vi "Measurement Logic.vi"() -> ()   [LabVIEW 2021, in "DAQmx Continuous Voltage Input.lvlib"]
uses:
  DAQmx Continuous Voltage Input.lvlib
  Measurement Configuration.ctl
  Measurement Results.ctl
  <vilib>/MeasurementLink/MeasurementLink Measurement Server/Measure Call Context/Measure Call Context.lvclass
  <vilib>/Utility/error.llb/DialogType.ctl
  Typedef/Analog Start.ctl
  Typedef/Analog Pause.ctl
  Typedef/Waveform.ctl
  <vilib>/DAQmx/read.llb/DAQmx Read (Analog 1D Wfm NChan NSamp).vi
  <vilib>/DAQmx/create/channels.llb/DAQmx Create Channel (AI-Voltage-Basic).vi
  <vilib>/DAQmx/configure/timing.llb/DAQmx Timing (Sample Clock).vi
  <vilib>/DAQmx/configure/task.llb/DAQmx Configure Logging (TDMS).vi
  <vilib>/DAQmx/configure/trigger.llb/DAQmx Start Trigger (Digital Edge).vi
  <vilib>/DAQmx/configure/trigger.llb/DAQmx Start Trigger (Time).vi
  <vilib>/DAQmx/configure/trigger.llb/DAQmx Start Trigger (Analog Edge).vi
  <vilib>/DAQmx/miscellaneous.llb/DAQmx Fill In Error Info.vi
  <resource>/objmgr/daqmx.rc
panel:
  out "measure call context out":refnum<class "Measure Call Context.lvclass">
  in  "measure call context in":refnum<class "Measure Call Context.lvclass">
  out "measurement results":T1
  in  "measurement configuration":T2={"Max Voltage"=5.0, "Min Voltage"=-5.0, "Terminal Configuration"=-1, "Sample Rate"=1000.0, "Number of Samples"=100, "Logging Mode"=10231, "TDMS File Path"="", "Trigger Tab Enum"=enum."No Trigger", "Analog Start str"="", "Digital Start Source str"="", "Digital Pause Source str"="", "Digital Start Trigger Edge"=10280, "Digital Pause Trigger Pause When"=10192, "Physical Channel str"="Dev1/ai0", "Sample Clock Source str"="OnboardClock", "Select Time Manually"=FALSE, "When str"="", "Analog Pause str"=""} {"Digital Pause Trigger Pause When" items=["High"=10192, "Low"=10214]; "Digital Start Trigger Edge" items=["Rising"=10280, "Falling"=10171]; "Logging Mode" items=["Off"=10231, "Log and Read"=15842]; "Terminal Configuration" items=["default"=-1, "RSE"=10083, "NRSE"=10078, "Differential"=10106, "Pseudodifferential"=12529]}
  # "Source: LabVIEW - examples\\DAQmx\\Analog Input\\Voltage - Continuous Input.vi"
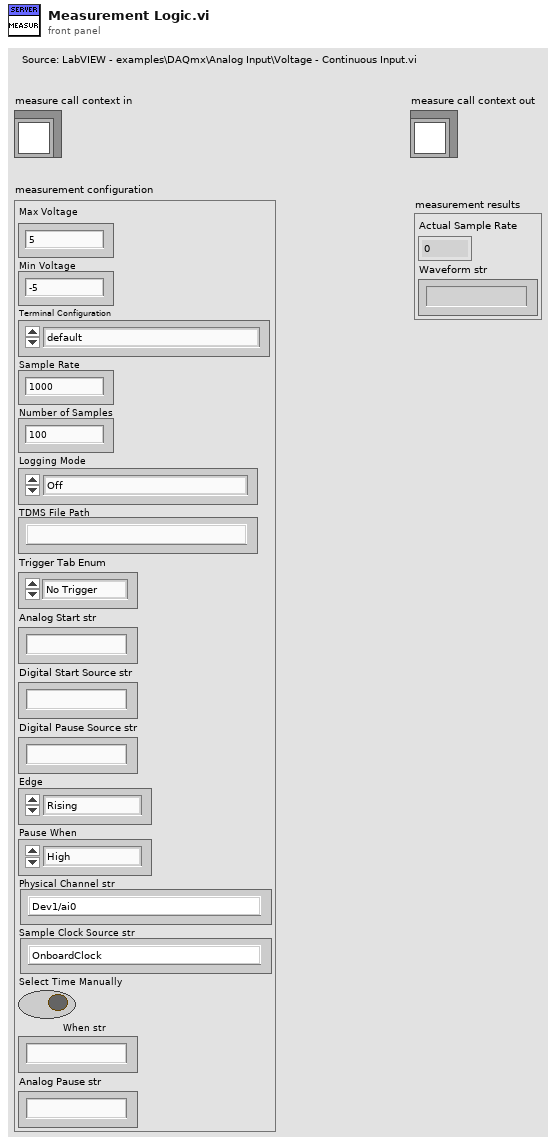
[diagram p1: front panel]
types:
  T1 = typedef "DAQmx Continuous Voltage Input.lvlib/Measurement Results.ctl" = cluster{"Actual Sample Rate":dbl, "Waveform str":string}
  T2 = typedef "DAQmx Continuous Voltage Input.lvlib/Measurement Configuration.ctl" = cluster{"Max Voltage":dbl, "Min Voltage":dbl, "Terminal Configuration":i32, "Sample Rate":dbl, "Number of Samples":i32, "Logging Mode":i32, "TDMS File Path":string, "Trigger Tab Enum":enum32{"No Trigger", "Digital Start", "Digital Pause", "Digital Reference", "Analog Start", "Analog Pause", "Analog Reference", "Time Start"}, "Analog Start str":string, "Digital Start Source str":string, "Digital Pause Source str":string, "Digital Start Trigger Edge":i32, "Digital Pause Trigger Pause When":i32, "Physical Channel str":string, "Sample Clock Source str":string, "Select Time Manually":bool, "When str":string, "Analog Pause str":string}
  T3 = typedef "DialogType.ctl" = u16
  T4 = enum32{"No Trigger", "Digital Start", "Digital Pause", "Digital Reference", "Analog Start", "Analog Pause", "Analog Reference", "Time Start"}
  T5 = typedef "DAQmx Continuous Voltage Input.lvlib/Analog Start.ctl" = cluster{"Analog Start Trigger Source":string, "Analog Start Trigger Slope":i32, "Analog Start Trigger Hysteresis":dbl, "Analog Start Trigger Level":dbl}
  T6 = typedef "DAQmx Continuous Voltage Input.lvlib/Analog Pause.ctl" = cluster{"Analog Pause Trigger Source":string, "Analog Pause Trigger Pause When":i32, "Analog Pause Trigger Level":dbl}
  T7 = typedef "DAQmx Continuous Voltage Input.lvlib/Waveform.ctl" = cluster{"Y":dbl[], "dt":dbl}
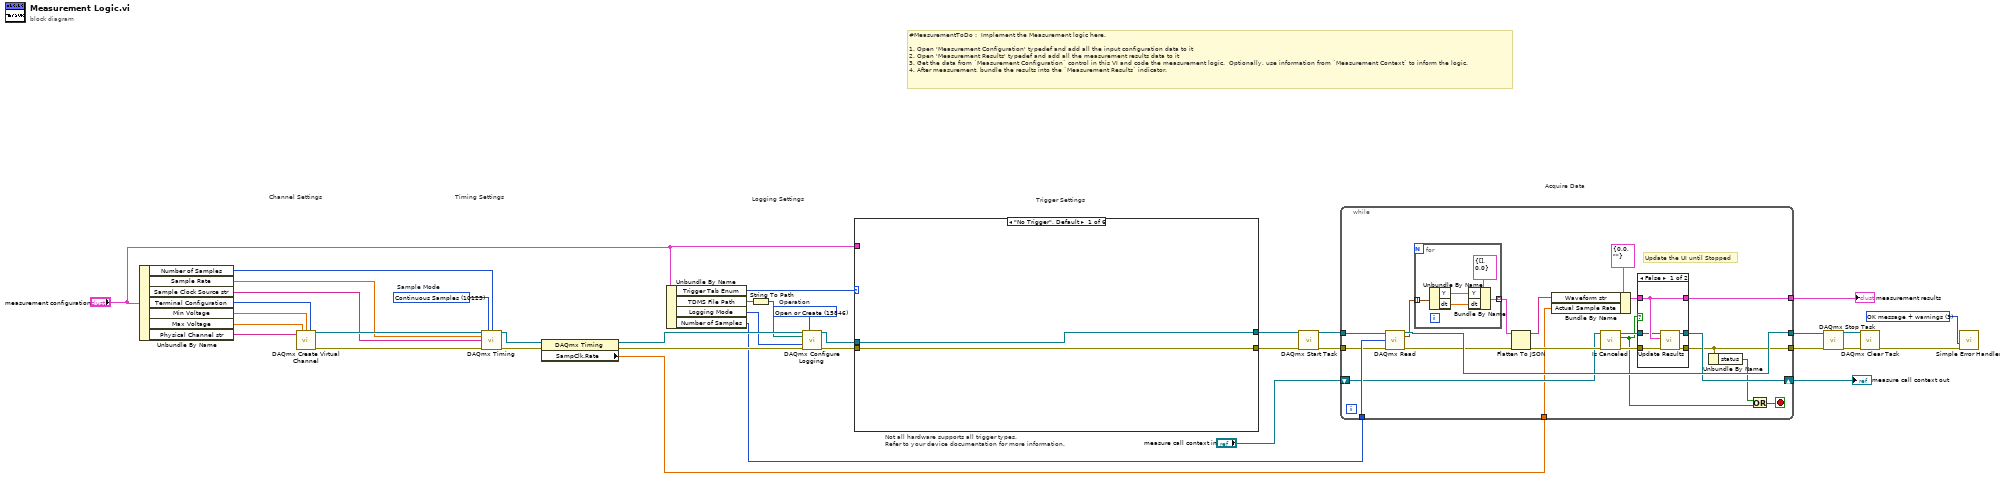
[diagram p0: block diagram]
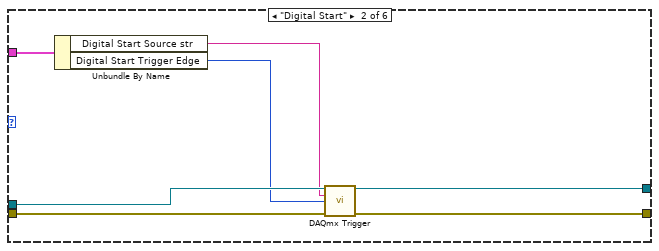
[diagram p2: hidden frame]
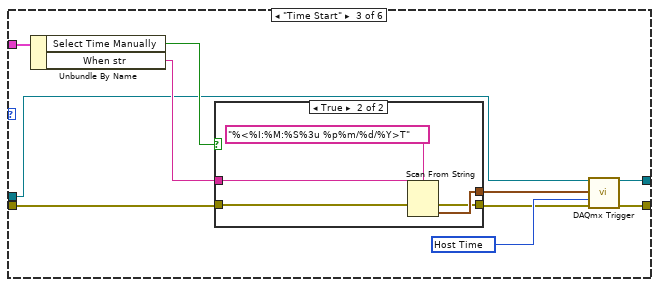
[diagram p3: hidden frame]
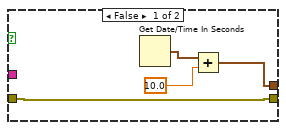
[diagram p4: hidden frame]
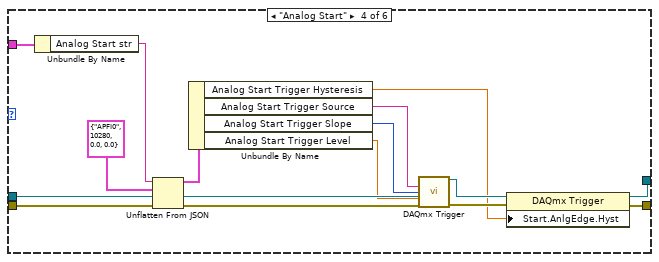
[diagram p5: hidden frame]
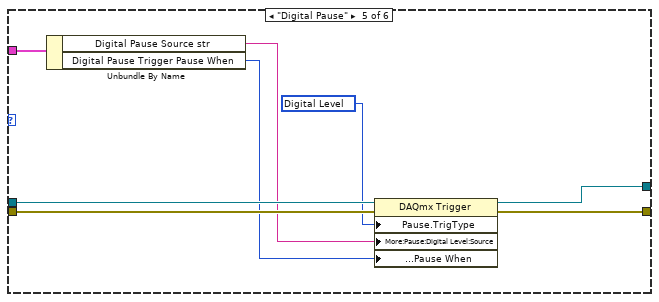
[diagram p6: hidden frame]
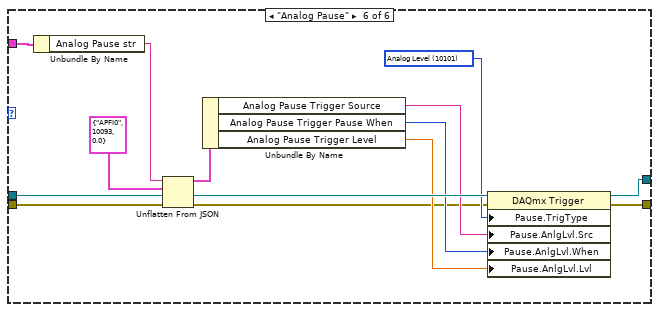
[diagram p7: hidden frame]
diagram:
  w22 = T3 3 items=["no dialog", "OK message", "continue or stop message", "OK message + warnings", "continue/stop + warnings"] ("type of dialog (OK msg:1)")
  w30 = 15846 items=["Open"=10437, "Open or Create"=15846, "Create or Replace"=15847, "Create"=15848]  # Operation
  w35 = 10123 items=["Finite Samples"=10178, "Continuous Samples"=10123, "Hardware Timed Single Point"=12522]  # Sample Mode
  # "Trigger Settings"
  # "Not all hardware supports all trigger types.\nRefer to your device documentation for more information."
  # "Acquire Data"
  # "Timing Settings"
  # "Channel Settings"
  # "Logging Settings"
  # "#MeasurementToDo :  Implement the Measurement logic here.\n\n1. Open 'Measurement Configuration' typedef and add all the input configuration data to it\n2. Open 'Measurement Results' typedef and add all the measurement results data to it\n3. Get the data from `Measurement Configuration` control in this VI and code the measurement logic.  Optionally, use information from `Measurement Context` to inform the logic.\n4. After measurement, bundle the results into the `Measurement Results` indicator."
  n1 = Unbundle By Name("measurement configuration") -> ("Number of Samples"=w13:i32, "Sample Rate"=w14:dbl, "Sample Clock Source str"=w5:string, "Terminal Configuration"=w15:i32, "Min Voltage"=w16:dbl, "Max Voltage"=w17:dbl, "Physical Channel str"=w6:string)
  n2 = call-poly <vilib>:"DAQmx Create Virtual Channel.vi"("maximum value"=w17, "minimum value"=w16, "input terminal configuration"=w15, "physical channels"=w6) -> ("task out"=w33:refnum<k21>, "error out"=w34:errorcluster)  [unwired: 10 in]
  n3 = call-poly <vilib>:"DAQmx Timing.vi"("task/channels in"=w33, "sample mode"=w35, "samples per channel"=w13, "rate"=w14, "source"=w5, "error in"=w34) -> ("task out"=w37:refnum<k21>, "error out"=w36:errorcluster)  [unwired: 8 in]
  n4 = property class="DAQmx Timing"(reference=w37, error in=w36) -> (reference out=w32:refnum<k21>, error out=w31:errorcluster, "SampClk.Rate"=w3:dbl)
  n5 = Unbundle By Name("measurement configuration") -> ("Trigger Tab Enum"=w1:T4, "TDMS File Path"=w11:string, "Logging Mode"=w10:i32, "Number of Samples"=w9:i32)
  n6 = String To Path(string=w11) -> (path=w12:path)
  n7 = call-poly <vilib>:"DAQmx Configure Logging.vi"("task/channels in"=w32, "operation"=w30, "file path"=w12, "logging mode"=w10, "error in"=w31) -> ("task out"=w21:refnum<k21>, "error out"=w2:errorcluster)  [unwired: 9 in]
  n8 = case shown="\"No Trigger\", Default" w1 {
    tunnel: w21 -> [w39 w46 w47 w80 w88 w101]
    tunnel: w2 -> [w38 w45 w50 w67 w85 w90]
    tunnel: [w39 w44 w56 w79 w87 w100] -> w19
    tunnel: [w38 w43 w55 w78 w86 w99] -> w20
    tunnel: "measurement configuration" -> [_ w42 w52 w75 w83 w97]
    frame "No Trigger", Default {
    }
    frame "Digital Start" {
      n9 = Unbundle By Name(w42) -> ("Digital Start Source str"=w41:string, "Digital Start Trigger Edge"=w40:i32)
      n10 = call-poly <vilib>:"DAQmx Trigger.vi"("task/channels in"=w46, "source"=w41, "edge"=w40, "error in"=w45) -> ("task out"=w44:refnum<k21>, "error out"=w43:errorcluster)  [unwired: 10 in]
    }
    frame "Time Start" {
      w54 = 16126 items=["Host Time"=16126, "I/O Device Time"=16127] ("timescale")
      n11 = Unbundle By Name(w52) -> ("Select Time Manually"=w51:bool, "When str"=w49:string)
      n12 = case shown="True" w51 {
        tunnel: [w58 w62] -> w53
        tunnel: w50 -> [w57 w63]
        tunnel: w49 -> [_ w64]
        tunnel: [w57 w61] -> w48
        frame False {
          n13 = Get Date/Time In Seconds() -> (seconds since 1Jan1904=w60:timestamp)
          n14 = Add(x=w60, y=10.0) -> (x+y=w58:timestamp)
        }
        frame True {
          n15 = Scan From String(format string="%<%I:%M:%S%3u %p%m/%d/%Y>T", input string=w64, error in=w63) -> (error out=w61:errorcluster, output 1=w62:timestamp)  [unwired: 2 in, 2 out]
        }
      }
      n16 = call-poly <vilib>:"DAQmx Trigger.vi"("task/channels in"=w47, "when"=w53, "timescale"=w54, "error in"=w48) -> ("task out"=w56:refnum<k21>, "error out"=w55:errorcluster)  [unwired: 10 in]
    }
    frame "Analog Start" {
      n17 = Unbundle By Name(w75) -> ("Analog Start str"=w74:string)
      n18 = Unflatten From JSON(JSON string=w74, type and defaults=T5 {"Analog Start Trigger Source"="APFI0", "Analog Start Trigger Slope"=10280, "Analog Start Trigger Hysteresis"=0.0, "Analog Start Trigger Level"=0.0} ("Analog Start"), error in (no error)=w67) -> (value=w72:T5, error out=w66:errorcluster)  [unwired: 4 in]
      n19 = Unbundle By Name(w72) -> ("Analog Start Trigger Hysteresis"=w71:dbl, "Analog Start Trigger Source"=w70:string, "Analog Start Trigger Slope"=w69:i32, "Analog Start Trigger Level"=w68:dbl)
      n20 = call-poly <vilib>:"DAQmx Trigger.vi"("task/channels in"=w80, "source"=w70, "slope"=w69, "level"=w68, "error in"=w66) -> ("task out"=w77:refnum<k21>, "error out"=w76:errorcluster)  [unwired: 9 in]
      n21 = property class="DAQmx Trigger"(reference=w77, error in=w76, "Start.AnlgEdge.Hyst"=w71) -> (reference out=w79:refnum<k21>, error out=w78:errorcluster)
    }
    frame "Digital Pause" {
      w84 = 10152 items=["Analog Level"=10101, "Analog Window"=10103, "Digital Level"=10152, "Digital Pattern"=10398, "None"=10230] ("Pause.TrigType")
      n22 = Unbundle By Name(w83) -> ("Digital Pause Source str"=w82:string, "Digital Pause Trigger Pause When"=w81:i32)
      n23 = property class="DAQmx Trigger"(reference=w88, error in=w85, "Pause.TrigType"=w84, "More:Pause:Digital Level:Source"=w82, "More:Pause:Digital Level:Pause When"=w81) -> (reference out=w87:refnum<k21>, error out=w86:errorcluster)
    }
    frame "Analog Pause" {
      w98 = 10101 items=["Analog Level"=10101, "Analog Window"=10103, "Digital Level"=10152, "Digital Pattern"=10398, "None"=10230] ("Pause.TrigType")
      n24 = Unbundle By Name(w97) -> ("Analog Pause str"=w96:string)
      n25 = Unflatten From JSON(JSON string=w96, type and defaults=T6 {"Analog Pause Trigger Source"="APFI0", "Analog Pause Trigger Pause When"=10093, "Analog Pause Trigger Level"=0.0} ("Analog Pause"), error in (no error)=w90) -> (value=w94:T6, error out=w89:errorcluster)  [unwired: 4 in]
      n26 = Unbundle By Name(w94) -> ("Analog Pause Trigger Source"=w93:string, "Analog Pause Trigger Pause When"=w92:i32, "Analog Pause Trigger Level"=w91:dbl)
      n27 = property class="DAQmx Trigger"(reference=w101, error in=w89, "Pause.TrigType"=w98, "Pause.AnlgLvl.Src"=w93, "Pause.AnlgLvl.When"=w92, "Pause.AnlgLvl.Lvl"=w91) -> (reference out=w100:refnum<k21>, error out=w99:errorcluster)
    }
  }
  n28 = call <vilib>:"DAQmx Start Task.vi"("task/channels in"=w19, "error in"=w20) -> ("task out"=w29:refnum<k21>, "error out"=w28:errorcluster)  [unwired: 12 in]
  n29 = while {
    tunnel: w29 -> [w122]
    tunnel: w28 -> [w113]
    tunnel: [w121] -> w26
    tunnel: [w112] -> w25
    tunnel: w9 -> [w120]
    tunnel: [w106] -> w7
    shift-right: [w114] -> w4
    shift-left: "measure call context in" -> [w107]
    tunnel: w3 -> [w102]
    stop <- w104 stop-if-true
    # "Update the UI until Stopped"
    n30 = call-poly <vilib>:"DAQmx Read.vi"("task/channels in"=w122, "number of samples per channel"=w120, "error in"=w113) -> ("task out"=w121:refnum<k21>, "data"=w119:waveform(dbl)[], "error out"=w109:errorcluster)  [unwired: 10 in]
    n31 = for {
      tunnel: w119 -> [w135] mode=indexing
      tunnel: [w131] -> w116 mode=indexing
      n32 = Unbundle By Name(w135) -> ("Y"=w133:dbl[], "dt"=w132:dbl)
      n33 = Bundle By Name(cluster=T7 {"Y"=[], "dt"=0.0} ("Waveform"), "Y"=w133, "dt"=w132) -> (w131:T7)
    }
    n34 = Flatten To JSON(anything=w116, error in (no error)=w109) -> (JSON string=w117:string, 11:w108:errorcluster)  [unwired: 1 in]
    n35 = Bundle By Name(cluster=T1 {"Actual Sample Rate"=0.0, "Waveform str"=""} ("Measurement Results"), "Waveform str"=w117, "Actual Sample Rate"=w102) -> (w115:T1)
    n36 = call <vilib>:"Is Canceled.vi"("error in"=w108, "measure call context in"=w107) -> ("error out"=w111:errorcluster, "is canceled?"=w103:bool, "measure call context out"=w110:refnum<class "Measure Call Context.lvclass">)  [unwired: 7 in]
    n37 = case shown="False" w103 {
      tunnel: w115 -> [w127 w130]
      tunnel: [w126 w129] -> w114
      tunnel: [w125 w128] -> w112
      tunnel: w111 -> [w124 w128]
      tunnel: w110 -> [w123 w129]
      tunnel: [w127 w130] -> w106
      frame False {
        n38 = call <vilib>:"Update Results.vi"("error in"=w124, "measurement results"=w127, "measure call context in"=w123) -> ("error out"=w125:errorcluster, "measure call context out"=w126:refnum<class "Measure Call Context.lvclass">)  [unwired: 7 in]
      }
      frame True {
      }
    }
    n39 = Unbundle By Name(w112) -> ("status"=w105:bool)
    n40 = Or(x=w105, y=w103) -> (x .or. y?=w104:bool)
  }
  "measurement results" <- w7
  "measure call context out" <- w4
  n41 = call <vilib>:"DAQmx Stop Task.vi"("task/channels in"=w26, "error in"=w25) -> ("task out"=w23:refnum<k21>, "error out"=w24:errorcluster)  [unwired: 12 in]
  n42 = call <vilib>:"DAQmx Clear Task.vi"("task in"=w23, "error in"=w24) -> ("error out"=w27:errorcluster)  [unwired: 13 in]
  n43 = call <vilib>:"Simple Error Handler.vi"("type of dialog (OK msg:1)"=w22, "error in (no error)"=w27) -> ()  [unwired: 3 in, 5 out]
